vi "IntakeStateMachine.vi"(8 "IntakeCancel":bool, 9 "HaveAlgaeSensor":bool, 10 "HaveCoralSensor":bool, 11 "IntakeCommands":bool[](array[boolean])) -> (0 "CurrentState":T1, 1 "RightMotorDemand":dbl, 2 "LeftMotorDemand":dbl, 3 "TopMotorDemand":dbl)   [LabVIEW 2023]
uses:
  IntakeStates.ctl
  <vilib>/Utility/semaphor.llb/Obtain Semaphore Reference.vi
  <vilib>/Rock Robotics/WPI/ThirdParty/JAS_Junk/TrajLib/Timer_Reset.vi
  <vilib>/Rock Robotics/WPI/ThirdParty/JAS_Junk/TrajLib/Trajectory_Library.lvlib
panel:
  # "Intake Coral"
  # "Intake Algae"
  # "Deposit Coral"
  # "Deposit Algae"
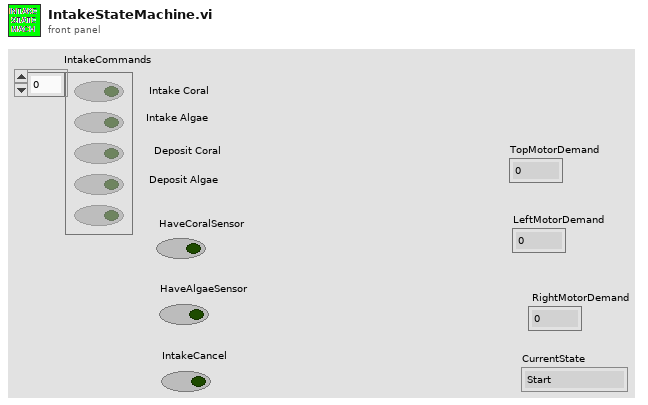
[diagram p1: front panel]
types:
  T1 = typedef "IntakeStates.ctl" = enum16{"Start", "WaitForCommand", "IntakeCoral", "IntakeAlgae", "WaitForCoral", "WaitForAlgae", "DepositCoral", "DepositAlgae", "DepositCoralTimer", "DepositAlgaeTimer"}
  T2 = typedef "Trajectory_Library.lvlib/TIMER.ctl" = cluster{"StartTime":dbl, "Accumulated TIme":dbl, "Running":bool, "semaphore":T3}
  T3 = typedef "Semaphore RefNum" = refnum<k1>
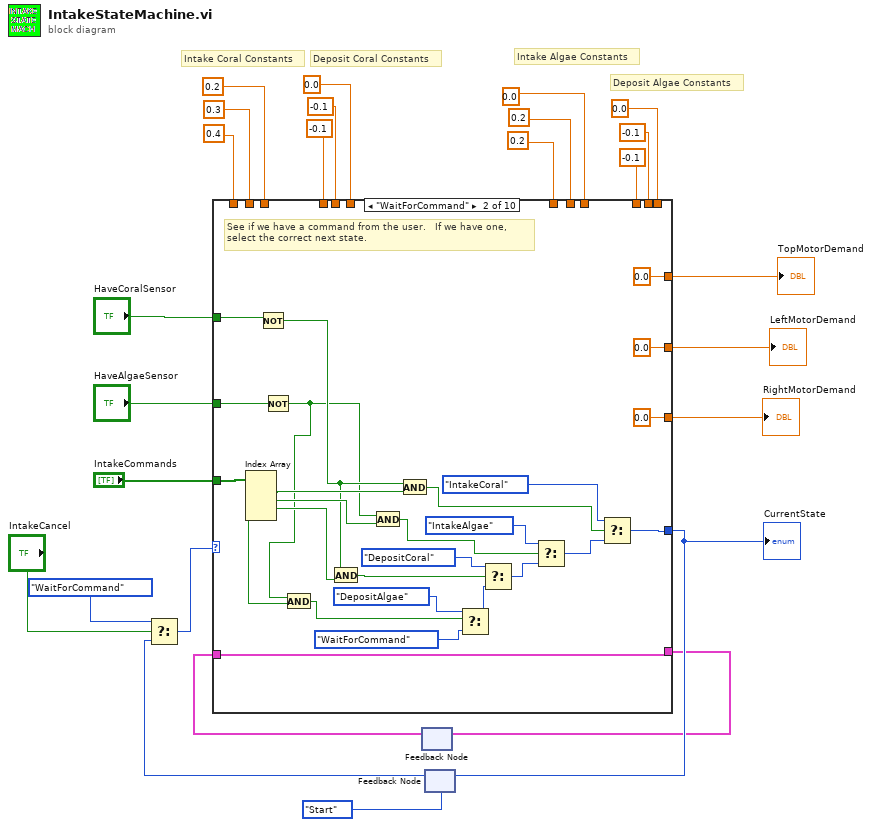
[diagram p0: block diagram]
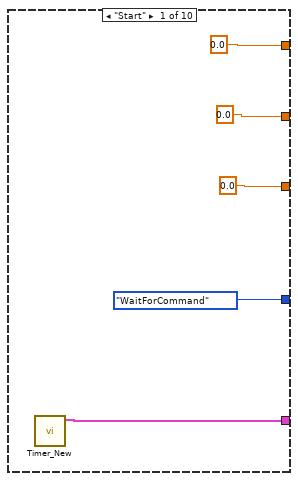
[diagram p2: hidden frame]
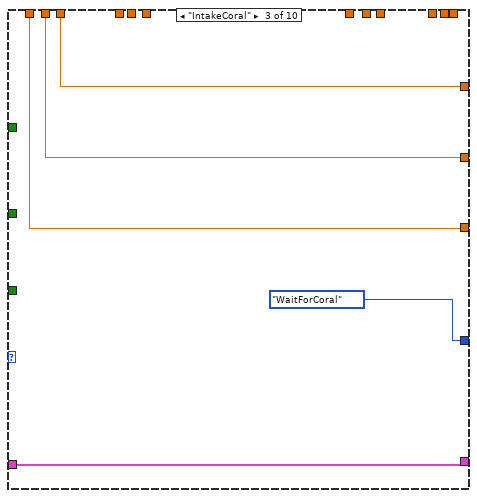
[diagram p3: hidden frame]
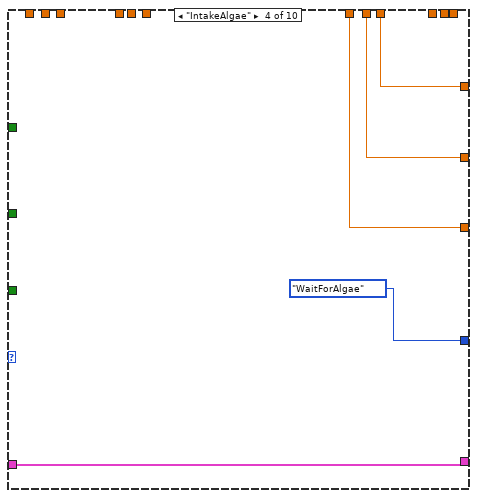
[diagram p4: hidden frame]
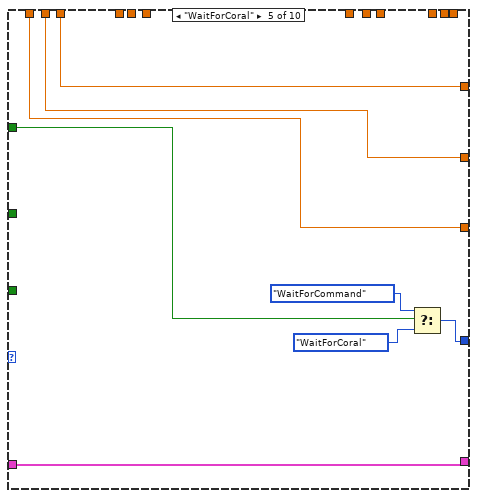
[diagram p5: hidden frame]
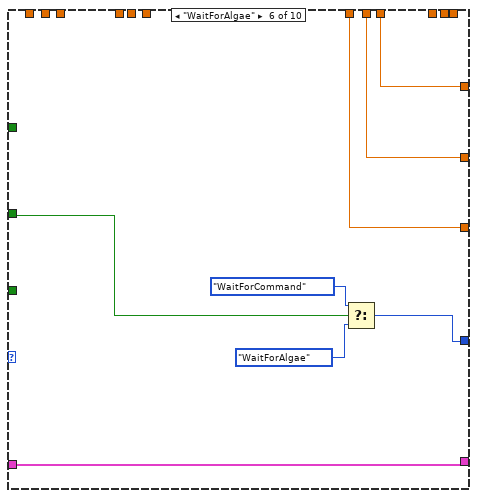
[diagram p6: hidden frame]
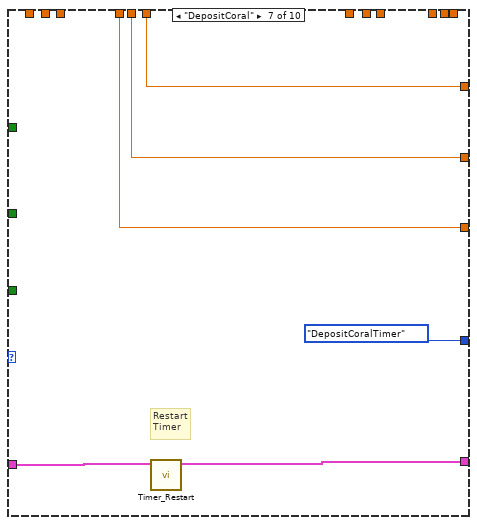
[diagram p7: hidden frame]
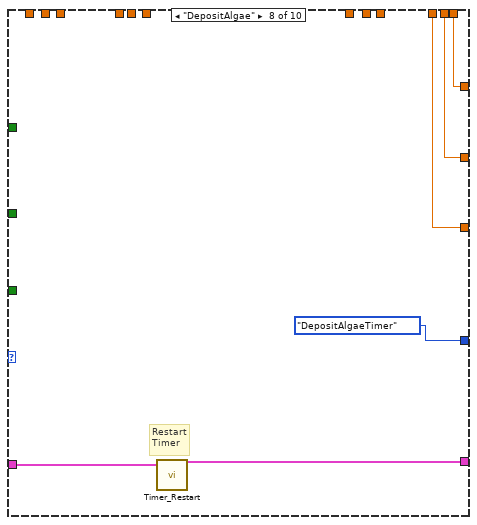
[diagram p8: hidden frame]
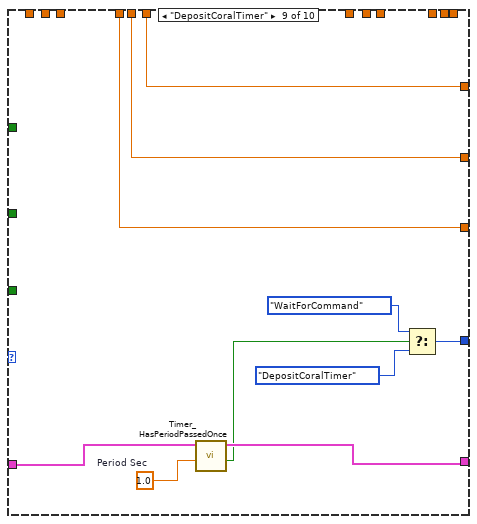
[diagram p9: hidden frame]
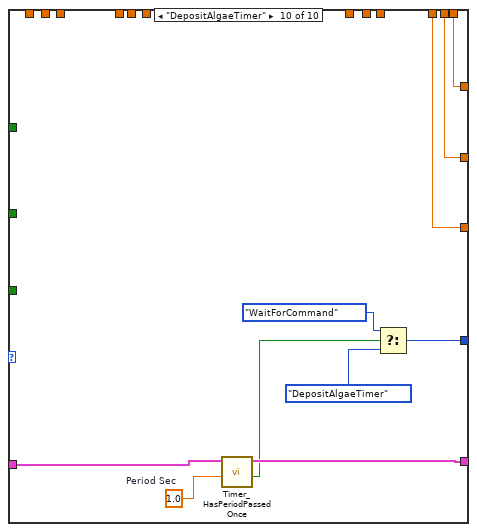
[diagram p10: hidden frame]
diagram:
  # "Deposit Algae Constants"
  # "Deposit Coral Constants"
  # "Intake Algae Constants"
  # "Intake Coral Constants"
  n1 = feedback #1() -> (w24:T2)  [unwired: 1 in]
  n2 = feedback #2(IntakeStates."Start" ("Enum 2")) -> (w3:T1)
  n3 = Select(t=IntakeStates."WaitForCommand", s="IntakeCancel", f=w3) -> (s? t:f=w2:T1)
  n4 = case shown="\"WaitForCommand\"" w2 {
    tunnel: [IntakeStates."WaitForCommand" w53 IntakeStates."WaitForCoral" ("Enum 2") IntakeStates."WaitForAlgae" ("Enum 2") w73 w81 IntakeStates."DepositCoralTimer" IntakeStates."DepositAlgaeTimer" w99 w112] -> w26
    tunnel: [w30 w57 w62 w67 w75 w80 w87 w94 w104 w114] -> w25
    tunnel: w24 -> [_ w57 w62 w67 w75 w80 w88 w95 w105 w115]
    tunnel: [0.0 ("TopMotorDemand") 0.0 ("TopMotorDemand") w61 w64 w70 w76 w86 w90 w98 w106] -> w23
    tunnel: [0.0 ("LeftMotorDemand") 0.0 ("LeftMotorDemand") w60 w65 w69 w77 w85 w91 w97 w107] -> w22
    tunnel: [0.0 ("RightMotorDemand") 0.0 ("RightMotorDemand") w59 w66 w68 w78 w84 w92 w96 w108] -> w21
    tunnel: "IntakeCommands" -> [_ w45 _ _ _ _ _ _ _ _]
    tunnel: "HaveCoralSensor" -> [_ w44 _ _ w71 _ _ _ _ _]
    tunnel: 0.2 -> [_ _ w61 _ w70 _ _ _ _ _]
    tunnel: 0.3 -> [_ _ w60 _ w69 _ _ _ _ _]
    tunnel: 0.4 -> [_ _ w59 _ w68 _ _ _ _ _]
    tunnel: 0.0 -> [_ _ _ w64 _ w76 _ _ _ _]
    tunnel: 0.2 -> [_ _ _ w65 _ w77 _ _ _ _]
    tunnel: 0.2 -> [_ _ _ w66 _ w78 _ _ _ _]
    tunnel: "HaveAlgaeSensor" -> [_ w33 _ _ _ w79 _ _ _ _]
    tunnel: -0.1 -> [_ _ _ _ _ _ w84 _ w96 _]
    tunnel: -0.1 -> [_ _ _ _ _ _ w85 _ w97 _]
    tunnel: 0.0 -> [_ _ _ _ _ _ w86 _ w98 _]
    tunnel: -0.1 -> [_ _ _ _ _ _ _ w92 _ w108]
    tunnel: -0.1 -> [_ _ _ _ _ _ _ w91 _ w107]
    tunnel: 0.0 -> [_ _ _ _ _ _ _ w90 _ w106]
    frame "Start" {
      n5 = call <vilib>:"Timer_New.vi"() -> ("TIMER"=w30:T2)  [unwired: 11 in]
    }
    frame "WaitForCommand" {
      # "See if we have a command from the user.   If we have one,\nselect the correct next state."
      n6 = Index Array(array=w45) -> (element #1=w43:bool, element #2=w41:bool, element #3=w39:bool, element #4=w35:bool)  [unwired: 4 in]
      n7 = Not(x=w44) -> (.not. x?=w36:bool)
      n8 = Not(x=w33) -> (.not. x?=w32:bool)
      n9 = And(x=w32, y=w35) -> (x .and. y?=w37:bool)
      n10 = And(x=w36, y=w39) -> (x .and. y?=w38:bool)
      n11 = And(x=w32, y=w41) -> (x .and. y?=w40:bool)
      n12 = And(x=w36, y=w43) -> (x .and. y?=w42:bool)
      n13 = Select(t=IntakeStates."DepositAlgae", s=w37, f=IntakeStates."WaitForCommand") -> (s? t:f=w47:T1)
      n14 = Select(t=IntakeStates."DepositCoral", s=w38, f=w47) -> (s? t:f=w50:T1)
      n15 = Select(t=IntakeStates."IntakeAlgae", s=w40, f=w50) -> (s? t:f=w52:T1)
      n16 = Select(t=IntakeStates."IntakeCoral", s=w42, f=w52) -> (s? t:f=w53:T1)
    }
    frame "IntakeCoral" {
    }
    frame "IntakeAlgae" {
    }
    frame "WaitForCoral" {
      n17 = Select(t=IntakeStates."WaitForCommand", s=w71, f=IntakeStates."WaitForCoral") -> (s? t:f=w73:T1)
    }
    frame "WaitForAlgae" {
      n18 = Select(t=IntakeStates."WaitForCommand", s=w79, f=IntakeStates."WaitForAlgae") -> (s? t:f=w81:T1)
    }
    frame "DepositCoral" {
      # "Restart\nTimer"
      n19 = call <vilib>:"Timer_Restart.vi"("in Timer"=w88) -> ("out Timer"=w87:T2)  [unwired: 10 in]
    }
    frame "DepositAlgae" {
      # "Restart\nTimer"
      n20 = call <vilib>:"Timer_Restart.vi"("in Timer"=w95) -> ("out Timer"=w94:T2)  [unwired: 10 in]
    }
    frame "DepositCoralTimer" {
      w103 = 1.0  # Period Sec
      n21 = call <vilib>:"Timer_HasPeriodPassedOnce.vi"("Period"=w103, "in Timer"=w105) -> ("Expired"=w101:bool, "out Timer"=w104:T2)  [unwired: 7 in, 1 out]
      n22 = Select(t=IntakeStates."WaitForCommand", s=w101, f=IntakeStates."DepositCoralTimer") -> (s? t:f=w99:T1)
    }
    frame "DepositAlgaeTimer" {
      w113 = 1.0  # Period Sec
      n23 = call <vilib>:"Timer_HasPeriodPassedOnce.vi"("Period"=w113, "in Timer"=w115) -> ("Expired"=w111:bool, "out Timer"=w114:T2)  [unwired: 7 in, 1 out]
      n24 = Select(t=IntakeStates."WaitForCommand", s=w111, f=IntakeStates."DepositAlgaeTimer") -> (s? t:f=w112:T1)
    }
  }
  "LeftMotorDemand" <- w22
  "RightMotorDemand" <- w21
  "TopMotorDemand" <- w23
  "CurrentState" <- w26
  n25 = feedback-in #1(w25) -> ()
  n26 = feedback-in #2(w26) -> ()
